vi "Display IMAQ at RPi Monitor.vi"() -> ()   [LabVIEW 2017]
uses:
  IMAQCV/LVOpenCV.lvlib
  IMAQCV/IMAQCV.lvlib
panel:
  in  "Display Delay ms":u32=10000
  out "error out":errorcluster
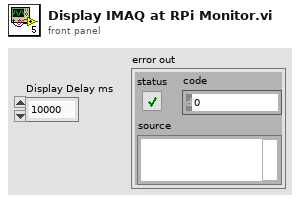
[diagram p1: front panel]
types:
  T1 = typedef "Image Type" = u32
  T2 = typedef "IMAQ Image.ctl" = refnum<image>
  T3 = typedef "IMAQCV.lvlib/IMAQCV Image.ctl" = refnum<vi>
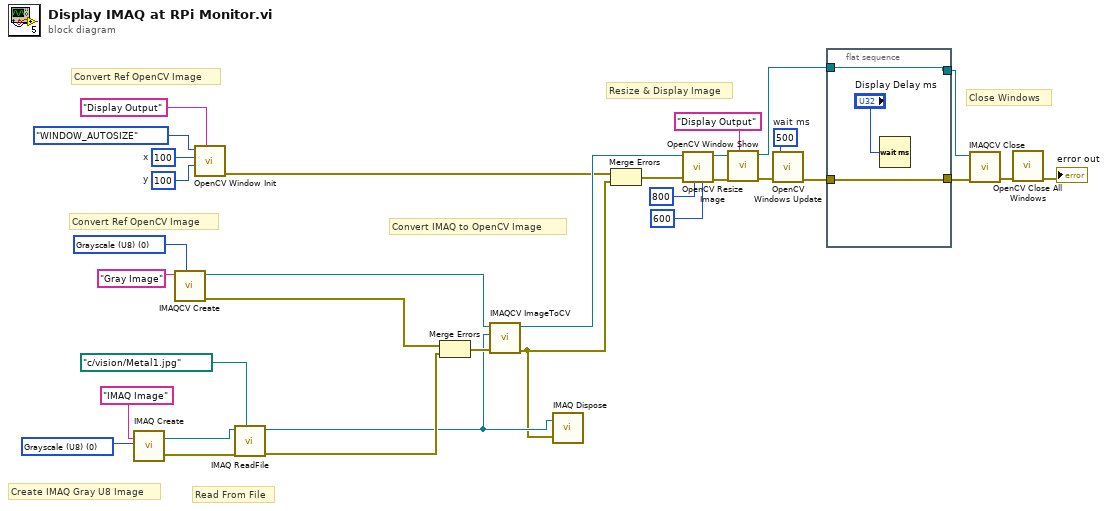
[diagram p0: block diagram]
diagram:
  w13 = 500  # wait ms
  w20 = u32 100  # y
  w21 = u32 100  # x
  w29 = T1 0 items=["Grayscale (U8)", "Grayscale (I16)", "Grayscale (SGL)", "Complex (CSG)", "RGB (U32)", "HSL (U32)", "RGB (U64)", "Grayscale (U16)"] ("Image Type")
  w24 = u32 0 items=["Grayscale (U8)", "Grayscale (I16)", "Grayscale (SGL)", "Complex (CSG)", "RGB (U32)", "HSL (U32)", "RGB (U64)", "Grayscale (U16)"] ("Image Type")
  # "Close Windows"
  # "Resize & Display Image"
  # "Convert Ref OpenCV Image"
  # "Convert Ref OpenCV Image"
  # "Convert IMAQ to OpenCV Image"
  # "Read From File"
  # "Create IMAQ Gray U8 Image"
  n1 = call "IMAQ Create"("Image Name"="IMAQ Image", "Image Type"=w29) -> ("New Image"=w31:T2, "error out"=w30:errorcluster)  [unwired: 2 in, 1 out]
  n2 = call "IMAQCV Create.vi"("Image Type"=w24, "Image Name"="Gray Image") -> ("error out"=w25:errorcluster, "Image Out"=w27:T3)  [unwired: 8 in]
  n3 = call "OpenCV Window Init.vi"("window name"="Display Output", "y"=w20, "x"=w21, "mode"=enum8{"WINDOW_AUTOSIZE", "WINDOW_FULLSCREEN"}."WINDOW_AUTOSIZE") -> ("error out"=w10:errorcluster)  [unwired: 7 in]
  n4 = call "IMAQ ReadFile"("File Path"=path "c:/vision/Metal1.jpg" ("appended path"), "error in (no error)"=w30, "Image"=w31) -> ("error out"=w3:errorcluster, "Image Out"=w2:T2)  [unwired: 2 in, 5 out]
  n5 = Merge Errors(w25, w3) -> (w26:errorcluster)
  n6 = call "IMAQCV ImageToCV.vi"("error in (no error)"=w26, "Variant In"=w2, "CV in"=w27) -> ("error out"=w1:errorcluster, "CV out"=w12:T3)  [unwired: 7 in]
  n7 = call "IMAQ Dispose"("Image"=w2, "error in (no error)"=w1) -> ()  [unwired: 4 in, 1 out]
  n8 = Merge Errors(w10, w1) -> (w11:errorcluster)
  n9 = call "OpenCV Resize Image.vi"("height"=u32 600, "width"=u32 800, "error in (no error)"=w11, "image in"=w12) -> ("error out"=w16:errorcluster, "image out"=w17:T3)  [unwired: 6 in]
  n10 = call "OpenCV Window Show.vi"("window name"="Display Output", "error in (no error)"=w16, "image in"=w17) -> ("error out"=w18:errorcluster, "image out"=w7:T3)  [unwired: 7 in]
  n11 = call "OpenCV Windows Update.vi"("error in (no error)"=w18, "wait ms"=w13) -> ("error out"=w9:errorcluster)  [unwired: 8 in, 1 out]
  n12 = flat-sequence {
    tunnel: [w36] -> w8
    tunnel: w9 -> [w36]
    tunnel: [w35] -> w6
    tunnel: w7 -> [w35]
    frame #0 {
      n13 = Wait (ms)(milliseconds to wait="Display Delay ms") -> ()  [unwired: 1 out]
    }
  }
  n14 = call "IMAQCV Close.vi"("error in (no error)"=w8, "Image"=w6) -> ("error out"=w5:errorcluster)  [unwired: 9 in]
  n15 = call "OpenCV Close All Windows.vi"("error in (no error)"=w5) -> ("error out"=→"error out":errorcluster)  [unwired: 10 in]
